vi "make_frame.vi"(0 "VIName":string, 1 "VIPath":string, 2 "id":string, 3 "type":string, 4 "label":string, 5 "parentId":string, 6 "properties":T2[](array[typedef]), 7 "metadata":T2[](array[typedef]), 9 "nodes":variant[](array[variant])) -> (14 "node":T1)   [LabVIEW 2020]
uses:
  node_var_property.ctl
  node.ctl
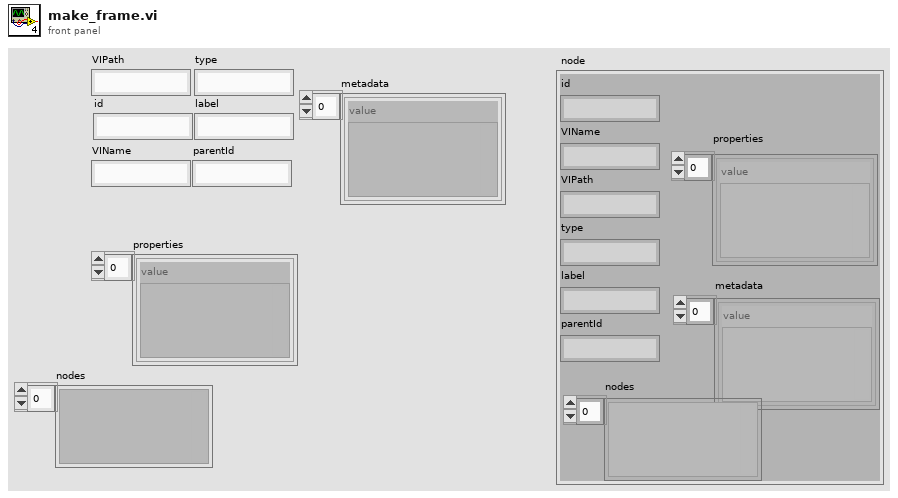
[diagram p1: front panel]
types:
  T1 = typedef "node.ctl" = cluster{"id":string, "VIName":string, "VIPath":string, "type":string, "label":string, "parentId":string, "properties":T2[], "metadata":T2[], "nodes":variant[]}
  T2 = typedef "node_var_property.ctl" = cluster{"value":variant}
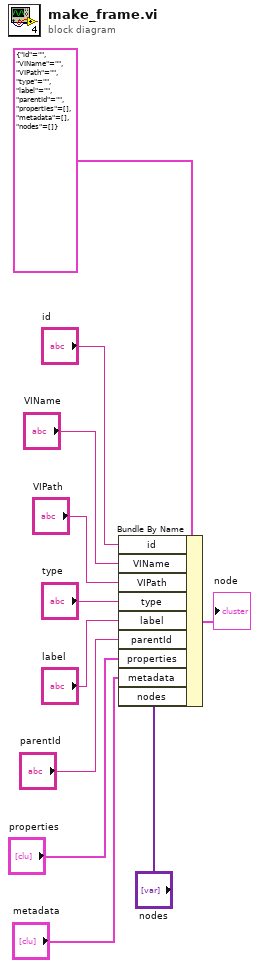
[diagram p0: block diagram]
diagram:
  n1 = Bundle By Name(cluster=T1 {"id"="", "VIName"="", "VIPath"="", "type"="", "label"="", "parentId"="", "properties"=[], "metadata"=[], "nodes"=[]} ("node_cluster"), "id"="id", "VIName"="VIName", "VIPath"="VIPath", "type"="type", "label"="label", "parentId"="parentId", "properties"="properties", "metadata"="metadata", "nodes"="nodes") -> (→"node":T1)
